vi "Save Recall Instr State.vi"(8 "error in (no error)":errorcluster, 9 "Setting Number (1:1)":u32(ring)=1 items=["0", "1", "2", "3", "4"], 10 "Mode (T:Recall)":bool=TRUE, 11 "VISA resource name":refnum<visa-resource-name>) -> (0 "error out":errorcluster, 3 "VISA resource name out":refnum<visa-resource-name>)   [LabVIEW 2010, in "Agilent 4194.lvlib"]
doc: "This function saves (recalls) the instrument state into (from) instrument memory."
uses:
  <instrlib>/Agilent 4194/Agilent 4194.lvlib
panel:
  # "Recall\nSave"
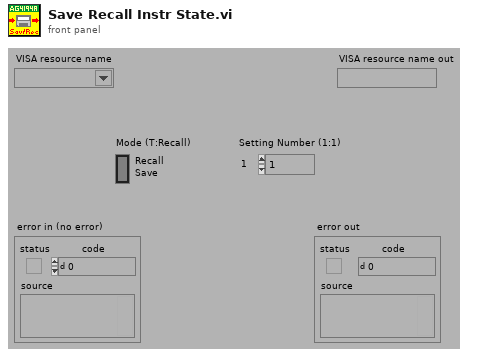
[diagram p1: front panel]
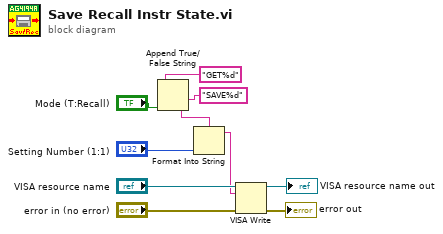
[diagram p0: block diagram]
diagram:
  n1 = Append True/False String(1:"Mode (T:Recall)", 2:"SAVE%d", 3:"GET%d") -> (0:w2:string)  [unwired: 1 in]
  n2 = Format Into String(format string=w2, "Setting Number (1:1)") -> (resulting string=w1:string)  [unwired: 2 in, 1 out]
  n3 = VISA Write(VISA resource name="VISA resource name", write buffer=w1, error in (no error)="error in (no error)") -> (VISA resource name out=→"VISA resource name out":refnum<visa-resource-name>, error out=→"error out":errorcluster)  [unwired: 1 out]
